vi "Error Message.vi"(0 "VISA resource name":refnum<visa-resource-name>, 11 "error in (no error)":errorcluster) -> (3 "Status":bool, 4 "VISA resource name out":refnum<visa-resource-name>, 8 "Error Code (0)":i32, 10 "Error Message (empty)":string, 15 "error out":errorcluster)   [LabVIEW 2010, in "Stanford Research PS300 Series.lvlib"]
doc: "This VI contains all the intrument specific error codes and descriptions. Use this VI after executing several instrument driver VIs to recognize and display any errors that may have occurred."
uses:
  <instrlib>/Stanford Research PS300 Series/Stanford Research PS300 Series.lvlib
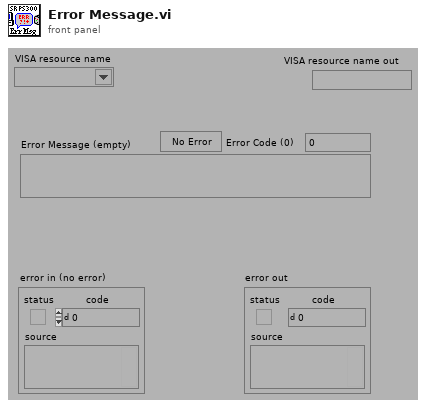
[diagram p1: front panel]
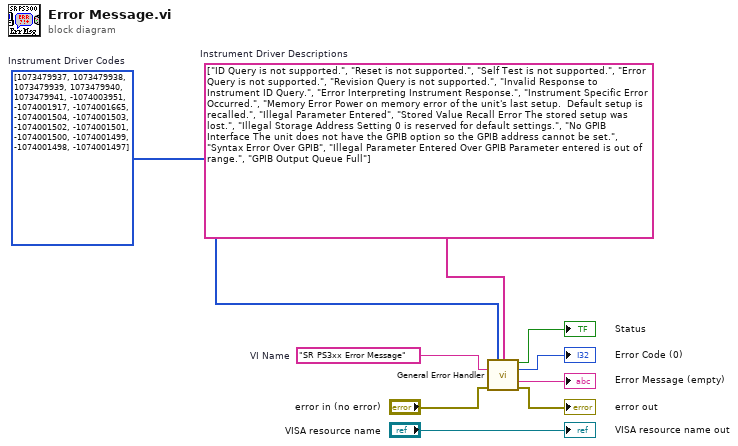
[diagram p0: block diagram]
diagram:
  w2 = i32[] [1073479937, 1073479938, 1073479939, 1073479940, 1073479941, -1074003951, -1074001917, -1074001665, -1074001504, -1074001503, -1074001502, -1074001501, -1074001500, -1074001499, -1074001498, -1074001497]  # Instrument Driver Codes
  w1 = string[] ["ID Query is not supported.", "Reset is not supported.", "Self Test is not supported.", "Error Query is not supported.", "Revision Query is not supported.", "Invalid Response to Instrument ID Query.", "Error Interpreting Instrument Response.", "Instrument Specific Error Occurred.", "Memory Error Power on memory error of the unit's last setup.  Default setup is recalled.", "Illegal Parameter Entered", "Stored Value Recall Error The stored setup was lost.", "Illegal Storage Address Setting 0 is reserved for default settings.", "No GPIB Interface The unit does not have the GPIB option so the GPIB address cannot be set.", "Syntax Error Over GPIB", "Illegal Parameter Entered Over GPIB Parameter entered is out of range.", "GPIB Output Queue Full"]  # Instrument Driver Descriptions
  w6 = "SR PS3xx Error Message"  # VI Name
  n1 = call <vilib>:"General Error Handler.vi"("[user-defined codes]"=w2, "[user-defined descriptions]"=w1, "[error source] (\" \")"=w6, "error in (no error)"="error in (no error)") -> ("error?"=→"Status":bool, "code out"=→"Error Code (0)":i32, "message"=→"Error Message (empty)":string, "error out"=→"error out":errorcluster)  [unwired: 7 in, 1 out]
  "VISA resource name out" <- "VISA resource name"
